vi "Correl Uneven LDA.vi"(9 "interp. method":i32(ring) items=["nearest", "linear", "spline", "cubic Hermite", "Lagrange"], 10 "Cluster 2":T2={"Colour"=0, "Inst type"=enum."Pitot-static tube", "Inst name"="Manometer voltage", "Symbol"="U", "Code name"="", "Extra Info"="U", "Inst Array"=enum."PWA", "Index"=0, "Voltage Index"=0, "Extra Titles"=[], "Extra Values"=[], "Eng Values"=[], "Time (ms)"=[], "TT / Voltage"=[], "u^2"=0.0, "U"=0.0, "u^3/(u^2)^(1.5)"=0.0, "u^4"=0.0, "u^4/(u^2)^2 -3"=0.0, "Mean % Err"=0.0, "% u'/U"=0.0} {"% u'/U" format="%.2f"; "Mean % Err" format="%.2f"; "u^4/(u^2)^2 -3" format="%.2f"; "u^4" format="%.2f"; "u^3/(u^2)^(1.5)" format="%.2f"; "U" format="%.2f"; "u^2" format="%.2f"}, 11 "Cluster 1":T2={"Colour"=0, "Inst type"=enum."Pitot-static tube", "Inst name"="Manometer voltage", "Symbol"="U", "Code name"="", "Extra Info"="U", "Inst Array"=enum."PWA", "Index"=0, "Voltage Index"=0, "Extra Titles"=[], "Extra Values"=[], "Eng Values"=[], "Time (ms)"=[], "TT / Voltage"=[], "u^2"=0.0, "U"=0.0, "u^3/(u^2)^(1.5)"=0.0, "u^4"=0.0, "u^4/(u^2)^2 -3"=0.0, "Mean % Err"=0.0, "% u'/U"=0.0} {"% u'/U" format="%.2f"; "Mean % Err" format="%.2f"; "u^4/(u^2)^2 -3" format="%.2f"; "u^4" format="%.2f"; "u^3/(u^2)^(1.5)" format="%.2f"; "U" format="%.2f"; "u^2" format="%.2f"}) -> (3 "Stats out":T1)   [LabVIEW 2011]
uses:
  Controls/Analysis_info_cluster.ctl
  Controls/Inst_type.ctl
  Controls/Instrument_Array.ctl
  <vilib>/gmath/NI_Gmath.lvlib
panel:
  out "Ref size":i32
  out "Interp size":i32
  out "T1 and T2 made coincident 2":cluster{"yi":dbl[], "yi":dbl[]}[](graph)
  out "U1 and U2 made coincident":cluster{"yi":dbl[], "yi":dbl[]}[](graph)
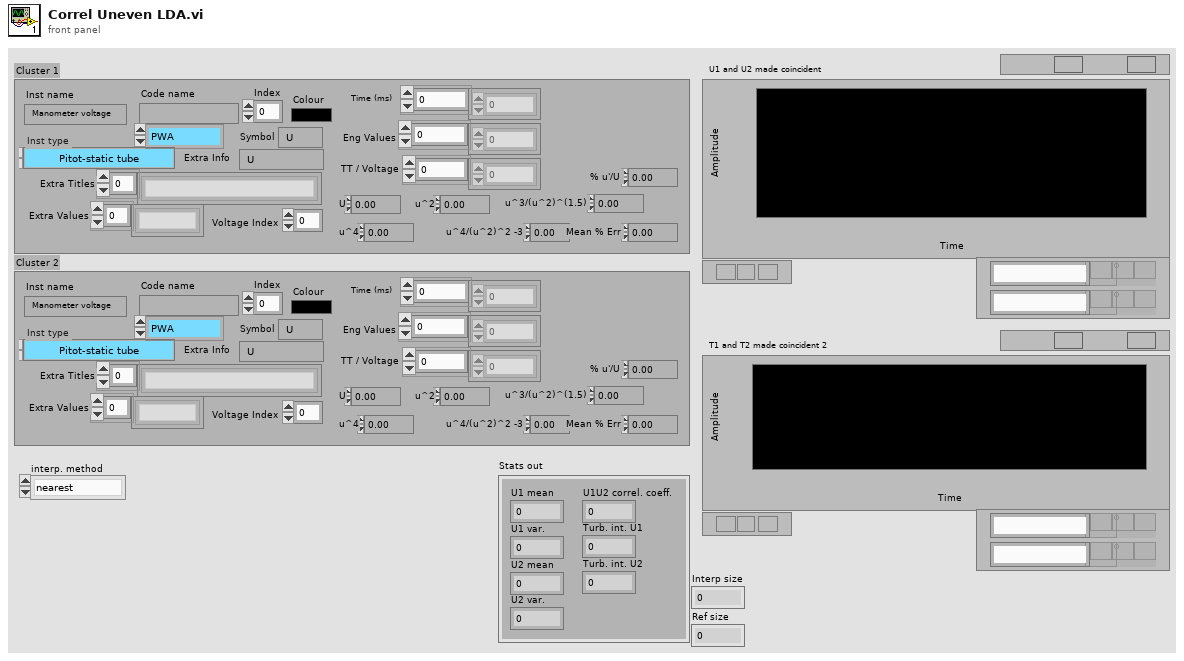
[diagram p1: front panel]
types:
  T1 = cluster{"U1 mean":dbl, "U1 var.":dbl, "U2 mean":dbl, "U2 var.":dbl, "U1U2 correl. coeff.":dbl, "Turb. int. U1":dbl, "Turb. int. U2":dbl}
  T2 = typedef "Analysis_info_cluster.ctl" = cluster{"Colour":u32, "Inst type":T3, "Inst name":string, "Symbol":string, "Code name":string, "Extra Info":string, "Inst Array":T4, "Index":i32, "Voltage Index":i32, "Extra Titles":string[], "Extra Values":string[], "Eng Values":dbl[], "Time (ms)":dbl[], "TT / Voltage":dbl[], "u^2":dbl, "U":dbl, "u^3/(u^2)^(1.5)":dbl, "u^4":dbl, "u^4/(u^2)^2 -3":dbl, "Mean % Err":dbl, "% u'/U":dbl}
  T3 = typedef "Inst_type.ctl" = enum16{"Propeller anemometer", "Raw voltage", "Pressure Transducer", "Pitot-static tube", "Preston tube", "Hot wire", "Cross wire 1", "Cross wire 2", "Generic Linear", "Generic Polynomial", "Generic BackPoly", "Fast FID", "Thermocouple", "Cold wire", "Pulsed Wire", "LDA Vel", "LDA Tran time", "LDA Arr time"}
  T4 = typedef "Instrument_Array.ctl" = enum16{"PWA", "LDA", "Analogue"}
  T5 = cluster{"Time (ms)":dbl[], "Eng Values":dbl[], "TT / Voltage":dbl[]}
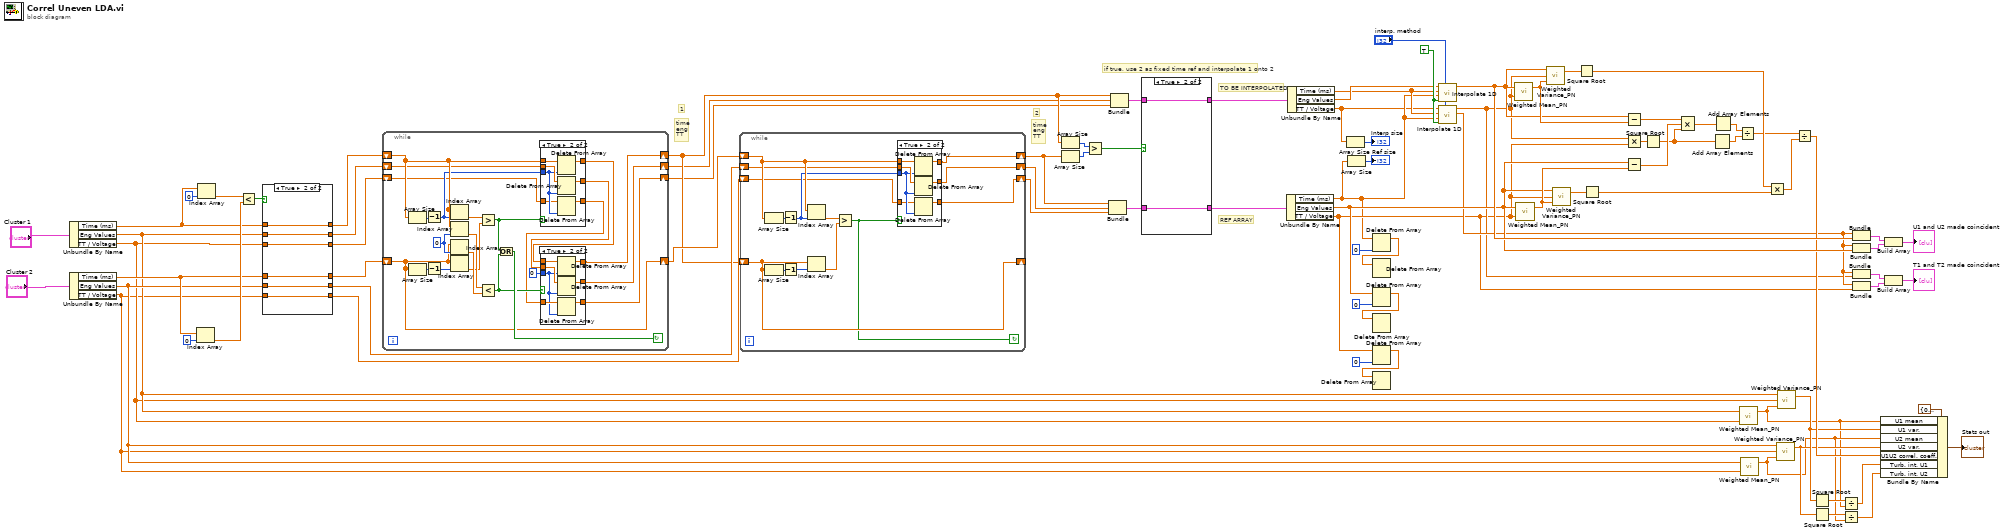
[diagram p0: block diagram]
diagram:
  w55 = TRUE ("X is monotonic")
  # "TO BE INTERPOLATED"
  # "REF ARRAY"
  # "if true, use 2 as fixed time ref and interpolate 1 onto 2"
  # "2"
  # "1"
  # "time\neng\nTT"
  # "time\neng\nTT"
  n1 = Unbundle By Name("Cluster 1") -> ("Time (ms)"=w77:dbl[], "Eng Values"=w25:dbl[], "TT / Voltage"=w7:dbl[])
  n2 = Unbundle By Name("Cluster 2") -> ("Time (ms)"=w72:dbl[], "Eng Values"=w26:dbl[], "TT / Voltage"=w6:dbl[])
  n3 = Index Array(array=w72, index=0) -> (element=w79:dbl)
  n4 = Index Array(array=w77, index=0) -> (element=w80:dbl)
  n5 = Less?(x=w80, y=w79) -> (x < y?=w78:bool)
  n6 = case shown="True" w78 {
    tunnel: w77 -> [w85 w96]
    tunnel: [w90 w96] -> w76
    tunnel: [w89 w95] -> w75
    tunnel: w25 -> [w86 w95]
    tunnel: [w88 w94] -> w74
    tunnel: w7 -> [w87 w94]
    tunnel: [w85 w93] -> w73
    tunnel: w72 -> [w90 w93]
    tunnel: [w86 w92] -> w70
    tunnel: w26 -> [w89 w92]
    tunnel: [w87 w91] -> w69
    tunnel: w6 -> [w88 w91]
    frame False {
    }
    frame True {
    }
  }
  n7 = while {
    shift-right: [w107] -> w63
    shift-left: w76 -> [w112]
    shift-right: [w106] -> w62
    shift-left: w75 -> [w111]
    shift-right: [w97] -> w71
    shift-left: w73 -> [w97]
    shift-right: [w98] -> w61
    shift-left: w74 -> [w100]
    stop <- w113 continue-if-true
    w119 = 0 ("index")
    n8 = Array Size(array=w112) -> (size(s)=w104:i32)
    n9 = Array Size(array=w97) -> (size(s)=w102:i32)
    n10 = Decrement(x=w104) -> (x-1=w103:i32)
    n11 = Decrement(x=w102) -> (x-1=w101:i32)
    n12 = Index Array(array=w112, index=w103) -> (element=w116:dbl)
    n13 = Index Array(array=w112, index=w119) -> (element=w118:dbl)
    n14 = Index Array(array=w97, index=w119) -> (element=w117:dbl)
    n15 = Index Array(array=w97, index=w101) -> (element=w115:dbl)
    n16 = Greater?(x=w116, y=w115) -> (0:w114:bool)
    n17 = Less?(x=w118, y=w117) -> (x < y?=w110:bool)
    n18 = Or(x=w114, y=w110) -> (x .or. y?=w113:bool)
    n19 = case shown="True" w114 {
      tunnel: w112 -> [w132 w138]
      tunnel: w111 -> [w131 w139]
      tunnel: w103 -> [_ w135]
      tunnel: [w132 w137] -> w109
      tunnel: [w131 w136] -> w108
      tunnel: [w130 w134] -> w99
      tunnel: w100 -> [w130 w133]
      frame False {
      }
      frame True {
        n20 = Delete From Array(array=w138, index=w135) -> (array with subset deleted=w137:dbl[])  [unwired: 1 in, 1 out]
        n21 = Delete From Array(array=w139, index=w135) -> (array with subset deleted=w136:dbl[])  [unwired: 1 in, 1 out]
        n22 = Delete From Array(array=w133, index=w135) -> (array with subset deleted=w134:dbl[])  [unwired: 1 in, 1 out]
      }
    }
    n23 = case shown="True" w110 {
      tunnel: w109 -> [w122 w128]
      tunnel: w108 -> [w121 w129]
      tunnel: 0 -> [_ w123]
      tunnel: [w122 w127] -> w107
      tunnel: [w121 w126] -> w106
      tunnel: w99 -> [w120 w125]
      tunnel: [w120 w124] -> w98
      frame False {
      }
      frame True {
        n24 = Delete From Array(array=w128, index=w123) -> (array with subset deleted=w127:dbl[])  [unwired: 1 in, 1 out]
        n25 = Delete From Array(array=w129, index=w123) -> (array with subset deleted=w126:dbl[])  [unwired: 1 in, 1 out]
        n26 = Delete From Array(array=w125, index=w123) -> (array with subset deleted=w124:dbl[])  [unwired: 1 in, 1 out]
      }
    }
  }
  n27 = while {
    shift-right: [w142] -> w64
    shift-left: w71 -> [w151]
    shift-right: [w141] -> w65
    shift-left: w70 -> [w150]
    shift-right: [w144] -> _
    shift-left: w63 -> [w144]
    shift-right: [w140] -> w66
    shift-left: w69 -> [w145]
    stop <- w143 continue-if-true
    n28 = Array Size(array=w151) -> (size(s)=w149:i32)
    n29 = Array Size(array=w144) -> (size(s)=w147:i32)
    n30 = Decrement(x=w149) -> (x-1=w148:i32)
    n31 = Decrement(x=w147) -> (x-1=w146:i32)
    n32 = Index Array(array=w151, index=w148) -> (element=w153:dbl)
    n33 = Index Array(array=w144, index=w146) -> (element=w152:dbl)
    n34 = Greater?(x=w153, y=w152) -> (0:w143:bool)
    n35 = case shown="True" w143 {
      tunnel: w151 -> [w156 w162]
      tunnel: w150 -> [w155 w163]
      tunnel: w148 -> [_ w159]
      tunnel: [w156 w161] -> w142
      tunnel: [w155 w160] -> w141
      tunnel: [w154 w158] -> w140
      tunnel: w145 -> [w154 w157]
      frame False {
      }
      frame True {
        n36 = Delete From Array(array=w162, index=w159) -> (array with subset deleted=w161:dbl[])  [unwired: 1 in, 1 out]
        n37 = Delete From Array(array=w163, index=w159) -> (array with subset deleted=w160:dbl[])  [unwired: 1 in, 1 out]
        n38 = Delete From Array(array=w157, index=w159) -> (array with subset deleted=w158:dbl[])  [unwired: 1 in, 1 out]
      }
    }
  }
  n39 = Array Size(array=w63) -> (size(s)=w68:i32)
  n40 = Array Size(array=w64) -> (size(s)=w67:i32)
  n41 = Greater?(x=w68, y=w67) -> (0:w1:bool)
  n42 = Bundle("Time (ms)"=w64, "Eng Values"=w65, "TT / Voltage"=w66) -> (w59:T5)  [unwired: 1 in]
  n43 = Bundle("Time (ms)"=w63, "Eng Values"=w62, "TT / Voltage"=w61) -> (w60:T5)  [unwired: 1 in]
  n44 = case shown="True" w1 {
    tunnel: w60 -> [w164 w166]
    tunnel: w59 -> [w165 w167]
    tunnel: [w164 w167] -> w57
    tunnel: [w165 w166] -> w58
    frame False {
    }
    frame True {
    }
  }
  n45 = Unbundle By Name(w57) -> ("Time (ms)"=w5:dbl[], "Eng Values"=w27:dbl[], "TT / Voltage"=w8:dbl[])
  n46 = Unbundle By Name(w58) -> ("Time (ms)"=w29:dbl[], "Eng Values"=w54:dbl[], "TT / Voltage"=w4:dbl[])
  n47 = Array Size(array=w4) -> (size(s)=→"Interp size":i32)
  n48 = Array Size(array=w5) -> (size(s)=→"Ref size":i32)
  n49 = Delete From Array(array=w5, index=0) -> (array with subset deleted=w35:dbl[])  [unwired: 1 in, 1 out]
  n50 = Delete From Array(array=w35) -> ()  [unwired: 2 in, 2 out]
  n51 = Delete From Array(array=w27, index=0) -> (array with subset deleted=w32:dbl[])  [unwired: 1 in, 1 out]
  n52 = Delete From Array(array=w32) -> ()  [unwired: 2 in, 2 out]
  n53 = Delete From Array(array=w8, index=0) -> (array with subset deleted=w31:dbl[])  [unwired: 1 in, 1 out]
  n54 = Delete From Array(array=w31) -> ()  [unwired: 2 in, 2 out]
  n55 = call <vilib>:"Interpolate 1D.vi"("method"="interp. method", "X is monotonic"=w55, "xi"=w5, "X"=w29, "Y"=w54) -> ("yi"=w28:dbl[])  [unwired: 1 in, 5 out]
  n56 = call <vilib>:"Interpolate 1D.vi"("method"="interp. method", "X is monotonic"=w55, "xi"=w5, "X"=w29, "Y"=w4) -> ("xi used"=w10:dbl[], "yi"=w9:dbl[])  [unwired: 1 in, 4 out]
  n57 = call "Weighted Mean_PN.vi"("weights"=w9, "1D data"=w28) -> ("Weighted mean"=w39:dbl)  [unwired: 1 in]
  n58 = call "Weighted Mean_PN.vi"("weights"=w8, "1D data"=w27) -> ("Weighted mean"=w50:dbl)  [unwired: 1 in]
  n59 = call "Weighted Variance_PN.vi"("Weighted mean"=w39, "weights"=w9, "1D data"=w28) -> ("Weighted variance"=w52:dbl)  [unwired: 1 in]
  n60 = call "Weighted Variance_PN.vi"("Weighted mean"=w50, "weights"=w8, "1D data"=w27) -> ("Weighted variance"=w53:dbl)  [unwired: 1 in]
  n61 = Square Root(x=w52) -> (sqrt(x)=w42:dbl)
  n62 = Square Root(x=w53) -> (sqrt(x)=w43:dbl)
  n63 = Subtract(x=w28, y=w39) -> (x-y=w49:dbl[])
  n64 = Multiply(x=w9, y=w8) -> (x*y=w51:dbl[])
  n65 = Subtract(x=w27, y=w50) -> (x-y=w48:dbl[])
  n66 = Square Root(x=w51) -> (sqrt(x)=w47:dbl[])
  n67 = Compound Arithmetic op=MULTIPLY(w49, w48, w47) -> (w46:dbl[])
  n68 = Add Array Elements(numeric array=w47) -> (sum=w44:dbl)
  n69 = Add Array Elements(numeric array=w46) -> (sum=w45:dbl)
  n70 = Divide(x=w45, y=w44) -> (x/y=w41:dbl)
  n71 = call "Weighted Mean_PN.vi"("weights"=w7, "1D data"=w25) -> ("Weighted mean"=w16:dbl)  [unwired: 1 in]
  n72 = call "Weighted Mean_PN.vi"("weights"=w6, "1D data"=w26) -> ("Weighted mean"=w17:dbl)  [unwired: 1 in]
  n73 = Multiply(x=w42, y=w43) -> (x*y=w40:dbl)
  n74 = call "Weighted Variance_PN.vi"("Weighted mean"=w17, "weights"=w6, "1D data"=w26) -> ("Weighted variance"=w18:dbl)  [unwired: 1 in]
  n75 = call "Weighted Variance_PN.vi"("Weighted mean"=w16, "weights"=w7, "1D data"=w25) -> ("Weighted variance"=w21:dbl)  [unwired: 1 in]
  n76 = Divide(x=w41, y=w40) -> (x/y=w24:dbl)
  n77 = Square Root(x=w21) -> (sqrt(x)=w20:dbl)
  n78 = Square Root(x=w18) -> (sqrt(x)=w19:dbl)
  n79 = Divide(x=w20, y=w16) -> (x/y=w15:dbl)
  n80 = Divide(x=w19, y=w17) -> (x/y=w14:dbl)
  n81 = Bundle("xi used"=w10, "yi"=w28) -> (w37:cluster{"xi used":dbl[], "yi":dbl[]})  [unwired: 1 in]
  n82 = Bundle("xi used"=w10, "Eng Values"=w27) -> (w38:cluster{"xi used":dbl[], "Eng Values":dbl[]})  [unwired: 1 in]
  n83 = Bundle("xi used"=w10, "yi"=w9) -> (w12:cluster{"xi used":dbl[], "yi":dbl[]})  [unwired: 1 in]
  n84 = Bundle("xi used"=w10, "TT / Voltage"=w8) -> (w11:cluster{"xi used":dbl[], "TT / Voltage":dbl[]})  [unwired: 1 in]
  n85 = Bundle By Name(cluster=T1 {"U1 mean"=0.9954718465953092, "U1 var."=0.004524585800250516, "U2 mean"=0.9741719326855783, "U2 var."=0.003210872651225289, "U1U2 correl. coeff."=0.8552243395452833, "Turb. int. U1"=0.0, "Turb. int. U2"=0.0} ("Stats out"), "U1 mean"=w16, "U1 var."=w21, "U2 mean"=w17, "U2 var."=w18, "U1U2 correl. coeff."=w24, "Turb. int. U1"=w15, "Turb. int. U2"=w14) -> (→"Stats out":T1)
  n86 = Build Array(w37, w38) -> (→"U1 and U2 made coincident":cluster{"xi used":dbl[], "Eng Values":dbl[]}[])
  n87 = Build Array(w12, w11) -> (→"T1 and T2 made coincident 2":cluster{"xi used":dbl[], "TT / Voltage":dbl[]}[])
